vi "microFPGA_close.vi"(11 "VISA resource name":refnum<visa-resource-name>="COM208") -> ()   [LabVIEW 2016]
panel:
  out "error out":errorcluster
  in  "error in (no error)":errorcluster
  # "choose the COM port"
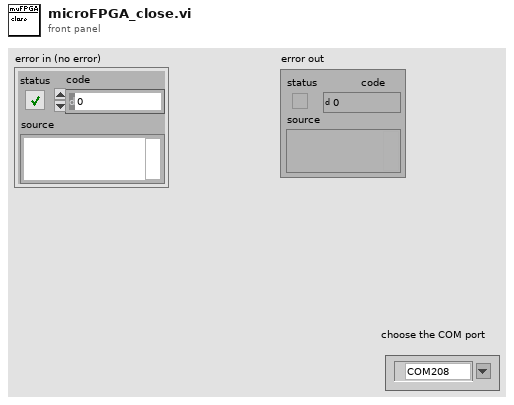
[diagram p1: front panel]
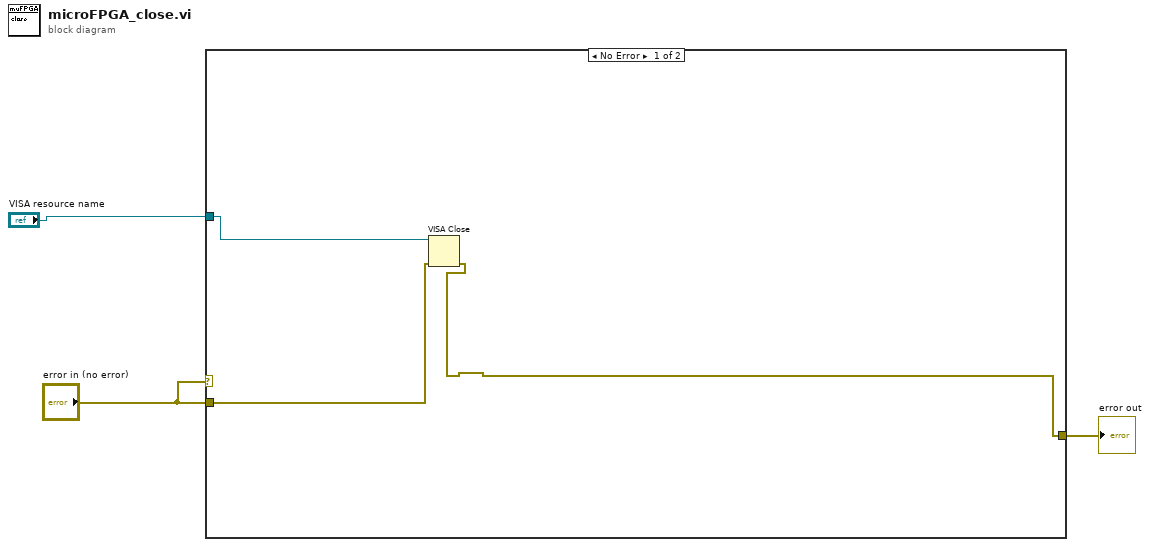
[diagram p0: block diagram]
diagram:
  n1 = case shown="No Error" "error in (no error)" {
    tunnel: "error in (no error)" -> [w5 w7]
    tunnel: [w4 w7] -> w3
    tunnel: "VISA resource name" -> [w6 _]
    frame No Error {
      n2 = VISA Close(VISA resource name=w6, error in (no error)=w5) -> (error out=w4:errorcluster)
    }
    frame Error {
    }
  }
  "error out" <- w3
